vi "Set ButtonGroupEnum By Ref.vi"(7 "ModeBtnRefs":refnum<vi>[](array[refnum]), 8 "error in":errorcluster, 11 "Boolean in":refnum<vi>) -> (0 "error out":errorcluster, 3 "Boolean out":refnum<vi>)   [LabVIEW 2017, in "ButtonGroupEnum.lvlib"]
doc: "Sets one button of a button group to TRUE and clears every other button in the group, so exactly one button is active."
uses:
  ButtonGroupEnum.lvlib
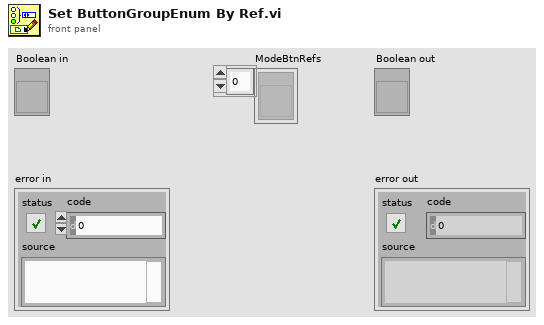
[diagram p1: front panel]
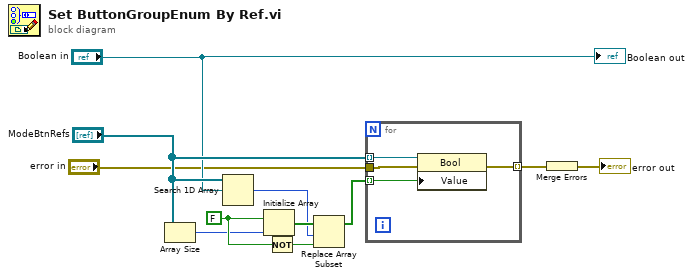
[diagram p0: block diagram]
diagram:
  w10 = FALSE
  n1 = Array Size(array="ModeBtnRefs") -> (size(s)=w9:i32)
  n2 = Search 1D Array(1D array="ModeBtnRefs", element="Boolean in") -> (index of element=w7:i32)  [unwired: 1 in]
  n3 = Initialize Array(w10, w9) -> (w8:bool[])
  n4 = Not(x=w10) -> (.not. x?=w6:bool)
  n5 = Replace Array Subset(array=w8, new element=w6, index=w7) -> (w5:bool[])
  n6 = for {
    tunnel: "ModeBtnRefs" -> [w15] mode=indexing
    tunnel: w5 -> [w14] mode=indexing
    tunnel: [w13] -> w4 mode=indexing
    tunnel: "error in" -> [w12]
    n7 = property class="Bool"(reference=w15, error in=w12, "Value"=w14) -> (error out=w13:errorcluster)  [unwired: 1 out]
  }
  n8 = Merge Errors(w4) -> (→"error out":errorcluster)
  "Boolean out" <- "Boolean in"
